vi "CRYString Array To Dotted Stirng.vi"(10 "String Array":string[](array[string])) -> (2 "Comma String":string)   [LabVIEW 2013]
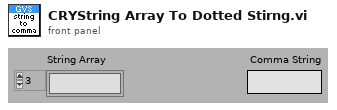
[diagram p1: front panel]
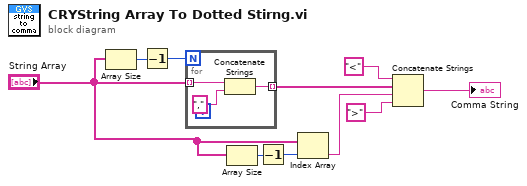
[diagram p0: block diagram]
diagram:
  n1 = Array Size(array="String Array") -> (size(s)=w9:i32)
  n2 = Decrement(x=w9) -> (x-1=w8:i32)
  n3 = for {
    N: w8 -> [_]
    tunnel: "String Array" -> [w13] mode=indexing
    tunnel: [w11] -> w10 mode=indexing
    n4 = Concatenate Strings(w13, "," ("string")) -> (w11:string)
  }
  n5 = Array Size(array="String Array") -> (size(s)=w6:i32)
  n6 = Decrement(x=w6) -> (x-1=w1:i32)
  n7 = Index Array(array="String Array", index=w1) -> (element=w5:string)
  n8 = Concatenate Strings("<" ("string"), w10, w5, ">" ("string")) -> (→"Comma String":string)
